vi "Configure Math.vi"(0 "VISA resource name":refnum<visa-resource-name>, 1 "Function (0: Volts)":u16(ring) items=["Volts", "Current", "Resistance", "Digitize Voltage", "Digitize Current"], 2 "Math Operation (1: Percent)":u16(ring)=1 items=["Y= mx+b", "Percent", "Reciprocal"], 3 "M Value (1)":dbl=1.0, 4 "B Value (0)":dbl, 5 "error in (no error)":errorcluster, 6 "Enable Math Function (T:Enable)":bool=TRUE, 7 "Percent Value (1)":dbl=1.0) -> (14 "VISA resource name out":refnum<visa-resource-name>, 19 "error out":errorcluster)   [LabVIEW 2021, in "Keithley 2450.lvlib"]
doc: "Configure the math operation performed by the instrument on collected data."
uses:
  <instrlib>/Keithley 2450/Keithley 2450.lvlib
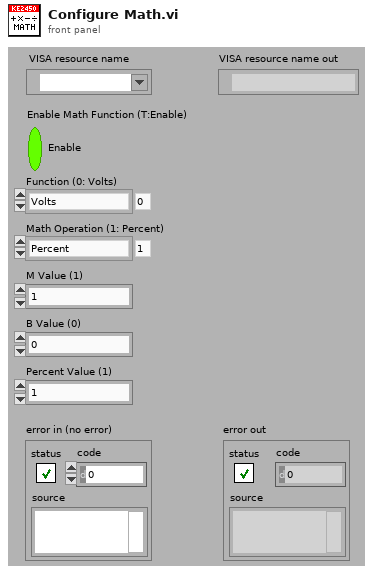
[diagram p1: front panel]
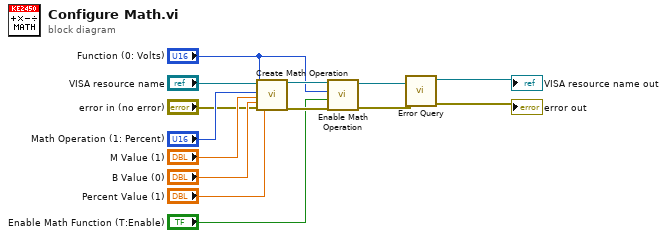
[diagram p0: block diagram]
diagram:
  n1 = call <instrlib>:"Create Math Operation.vi"("VISA resource name"="VISA resource name", "Function (0: Volts)"="Function (0: Volts)", "Math Operation (1: Percent)"="Math Operation (1: Percent)", "M Value (0)"="M Value (1)", "B Value (1)"="B Value (0)", "error in (no error)"="error in (no error)", "Percent Value (1)"="Percent Value (1)") -> ("VISA resource name out"=w14:refnum<visa-resource-name>, "error out"=w13:errorcluster)  [unwired: 11 in]
  n2 = call <instrlib>:"Enable Math Operation.vi"("error in (no error)"=w13, "Enable Math Operations (F:Disable)"="Enable Math Function (T:Enable)", "Function (0: Volts)"="Function (0: Volts)", "VISA resource name"=w14) -> ("error out"=w3:errorcluster, "VISA resource name out"=w4:refnum<visa-resource-name>)  [unwired: 6 in]
  n3 = call <instrlib>:"Error Query.vi"("error in (no error)"=w3, "VISA resource name"=w4) -> ("error out"=→"error out":errorcluster, "VISA resource name out"=→"VISA resource name out":refnum<visa-resource-name>)  [unwired: 6 in, 2 out]
